vi "ExecutionView(CSM).vi"(7 "Name(\"\" to use uuid)":string="TestStandOI") -> ()   [LabVIEW 2020, in "CSMScript-Engine(Lite).lvlib"]
doc: "------------- lvcsm -------------\n[CSMStates]\nItem 0 = \"Idle\"\nItem 1 = \"CSM Documentation\"\nItem 2 = \"Error Handler\"\nItem 3 = \"VI Reference\"\nItem 4 = \"Critical Error\"\nItem 5 = \"Target Timeout Error\"\nItem 6 = \"Target Error\"\nItem 7 = \"Async Response\"\nItem 8 = \"Response\"\nItem 9 = \"Async Message Posted\"\nItem 10 = \"Initialize Core Data\"\nItem 11 = \"Exit\"\nItem 12 = \"Data: Initialize\"\nItem 13 = \"Data: Get Configuration\"\nItem 14 = \"Data: Get Internal Data\"\nItem 15 = \"Data: Set Configuration\"\nItem 16 = \"Data: Cleanup\"\nItem 17 = \"UI: Initialize\"\nItem 18 = \"UI: Cursor Set\"\nItem 19 = \"UI: Front Panel State\"\nItem 20 = \"Macro: Initialize\"\nItem 21 = \"Macro: Exit\"\nItem 22 = \"TS: Load Sequence\"\nItem 23 = \"TS: Link to Engine\"\nItem 24 = \"TS: Test Started Handler\"\nItem 25 = \"TS: Step Start Handler\"\nItem 26 = \"TS: Step Complete Handler\"\nItem 27 = \"TS: Test Complete Handler\"\nItem 28 = \"Internal: action1\"\nItem 29 = \"Internal: action2\"\n\n[CSMStatus]\nItem 0 = \"Error Occurred@Error Handler\""
uses:
  CSMScript-Engine(Lite).lvlib
  <vilib>/Utility/miscctls.llb/LVRowAndColumnTypeDef.ctl
  Engine/Typedef/Def-StepComplete Event Data.ctl
  49887391-5aaa-4a15-bec5-64cc18cfe9d0.vi
  d29669de-e3bc-4aa1-abb6-bef5024a48d5.vi
  844f5a0a-3cc9-4d1a-ab8e-12611138b1fa.vi
  f99f0b71-739f-43a4-ba27-9b21da8a90fc.vi
  <userlib>/_NEVSTOP/Communicable State Machine(CSM)/_Support/Common/Format Timestamp.vi
  <userlib>/_NEVSTOP/Communicable State Machine(CSM)/AdvanceAPI/CSM - Revert Arguments-Safe String.vi
  <userlib>/_NEVSTOP/Communicable State Machine(CSM)/AdvanceAPI/CSM - Make String Arguments Safe.vi
  <userlib>/_NEVSTOP/Communicable State Machine(CSM)/AdvanceAPI/CSM - Break Down Multiple States String.vi
  <userlib>/_NEVSTOP/Communicable State Machine(CSM)/AdvanceAPI/CSM - Compact Multiple States.vi
  <userlib>/_NEVSTOP/Communicable State Machine(CSM)/_Support/GlobalEvent/GEvt-Generate with Rule Check.vi
  <userlib>/_NEVSTOP/Communicable State Machine(CSM)/_Support/GlobalEvent/Cache-GEvt Refs.vi
  <userlib>/_NEVSTOP/Communicable State Machine(CSM)/AdvanceAPI/CSM - Keywords.vi
  <userlib>/_NEVSTOP/Communicable State Machine(CSM)/_Support/ChangeFlag/FlagInstance-GEvt Refs.vi
  <userlib>/_NEVSTOP/Communicable State Machine(CSM)/_Support/ChangeFlag/ChangeFlag-Read.vi
  <userlib>/_NEVSTOP/Communicable State Machine(CSM)/_Shared/Trim Single-line Text.vi
  <userlib>/_NEVSTOP/Communicable State Machine(CSM)/_Support/ChangeFlag/ChangeFlagDB.vi
  <userlib>/_NEVSTOP/Communicable State Machine(CSM)/_Support/GlobalEvent/FGV-GlobalEventRef(lvlibp).vi
  <userlib>/_NEVSTOP/Communicable State Machine(CSM)/_Support/GlobalEvent/FGV-GlobalEventQueues(lvlibp).vi
  <userlib>/_NEVSTOP/Communicable State Machine(CSM)/_Support/GlobalEvent/GEvt-Valid Subscribers.vi
  <userlib>/_NEVSTOP/Communicable State Machine(CSM)/_Support/GlobalEvent/LogFilter/LogFilter - Check.vi
  <userlib>/_NEVSTOP/Communicable State Machine(CSM)/addons/API-String-Arugments-Support/_Support/Query Data as API String Arguments(variant).vi
  <userlib>/_NEVSTOP/Communicable State Machine(CSM)/addons/API-String-Arugments-Support/_Support/Convert API String Arguments to Data(variant).vi
  resource/global-rc-strings.vi
  <userlib>/_NEVSTOP/Communicable State Machine(CSM)/_Polymophic/CSM - Replace Marks in Messages.vi
  <userlib>/_NEVSTOP/Communicable State Machine(CSM)/_Support/GlobalEvent/LogFilter/LogFilter.lvclass
  <userlib>/_NEVSTOP/Communicable State Machine(CSM)/Communicable State Machine.lvlib
  <userlib>/_NEVSTOP/Communicable State Machine(CSM)/_tool/_ui/csm-ui-support.lvlib
panel:
  in  "Sequence Viewer":i32(listbox)=-1
  out "State History":string="[14:36:06.041] UI: Initialize\r[14:36:06.041] Initialize Core Data\r[14:36:06.041] Data: Initialize\r[14:36:06.041] Macro: Initialize\r"
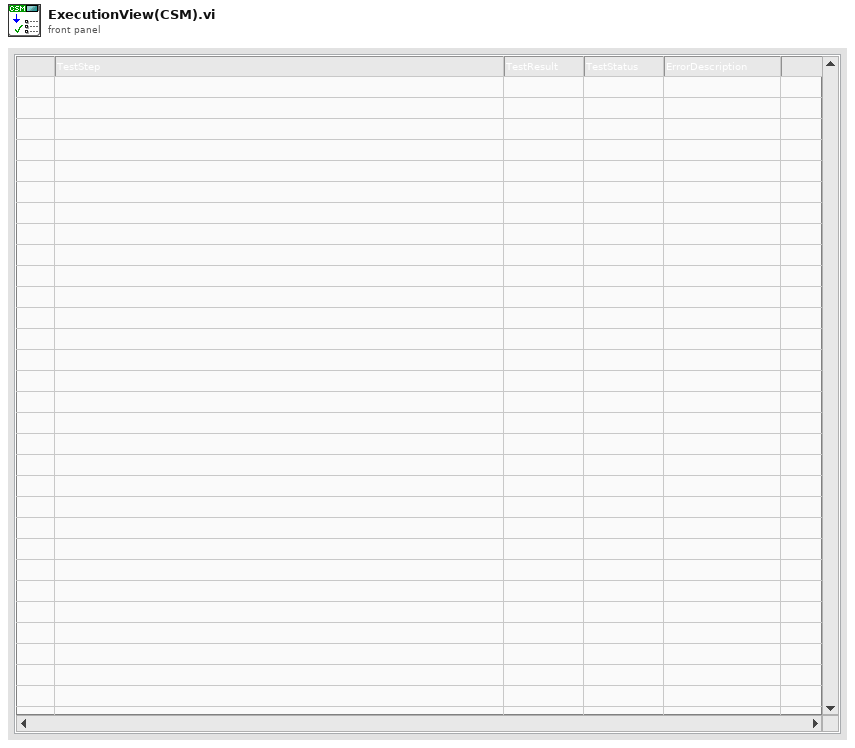
[diagram p1: front panel]
types:
  T1 = enum32{"Invalid", "Standard", "Closed", "Hidden", "Minimized", "Maximized"}
  T2 = enum32{"invalid app kind", "Development System", "Run Time System", "Student Edition", "Embedded LabVIEW", "Evaluation", "Custom"}
  T3 = typedef "LVRowAndColumnTypeDef.ctl" = cluster{"Row":i32, "Column":i32}
  T4 = typedef "CSMScript-Engine(Lite).lvlib/Def-StepComplete Event Data.ctl" = cluster{"index":i32, "Response":string, "error":errorcluster}
  T5 = typedef "Communicable State Machine.lvlib/_CSM_Response Source Message.ctl" = cluster{"‘State":string, "’Arguments":string, "’Error":errorcluster}
  T6 = cluster{"Current VI Reference":refnum<vi>, "Close Panel on Exit?":bool}
  T7 = cluster{"Core":cluster{"Current VI Reference":refnum<vi>, "Close Panel on Exit?":bool}, "Sequence Viewer":refnum<vi>, "ResponseMaxLen":i32}
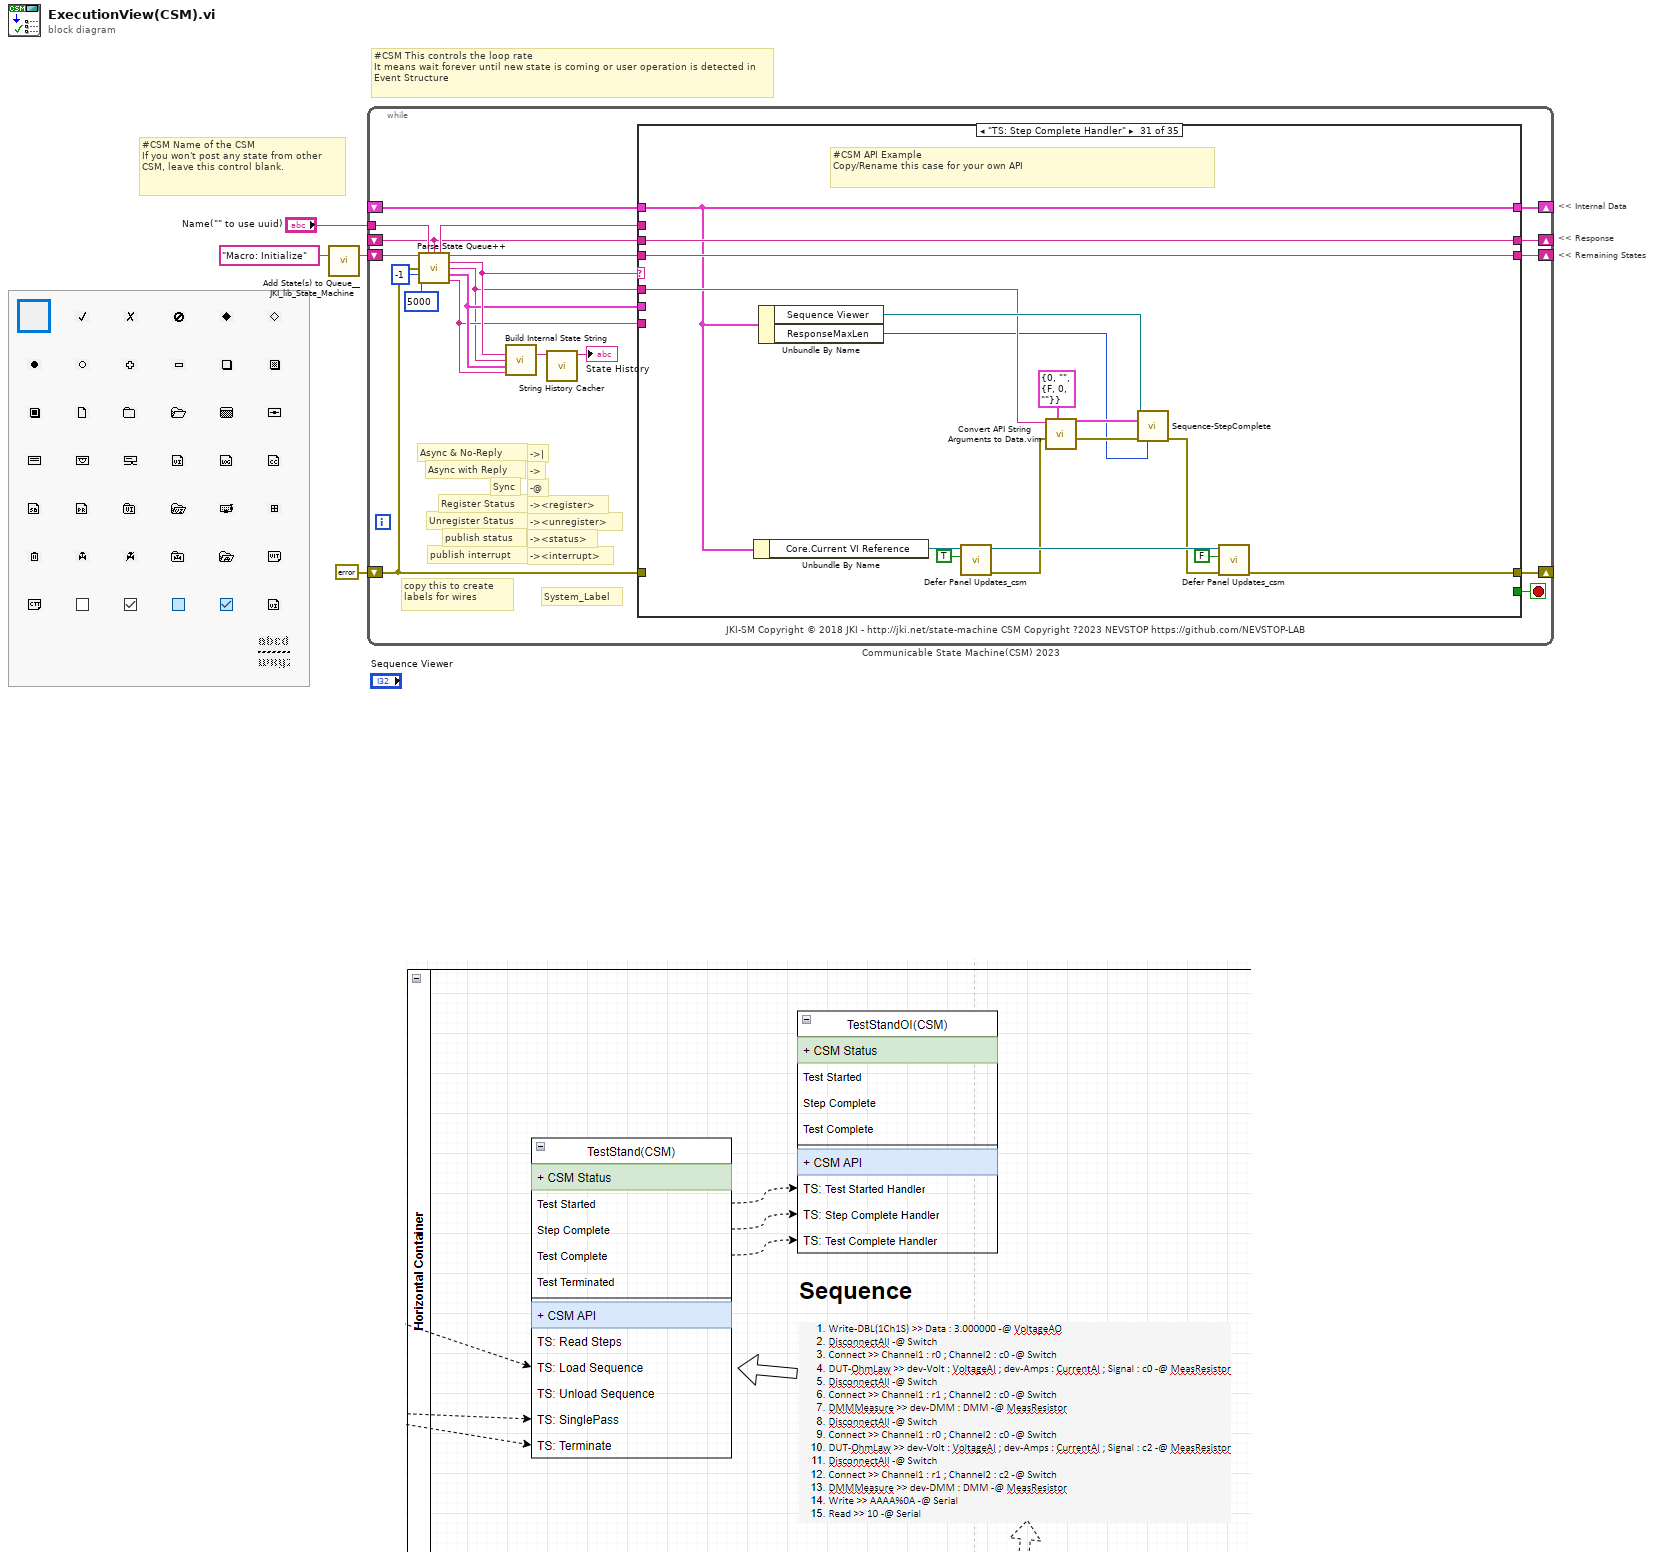
[diagram p0: block diagram]
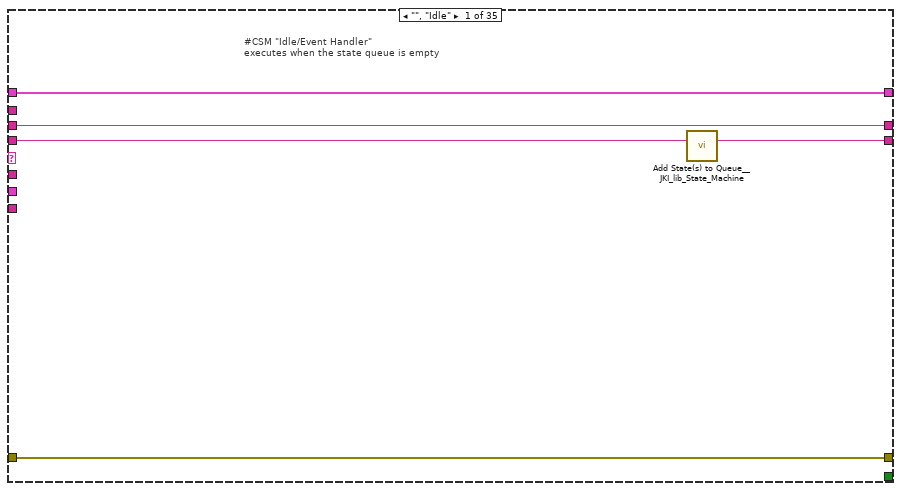
[diagram p2: hidden frame]
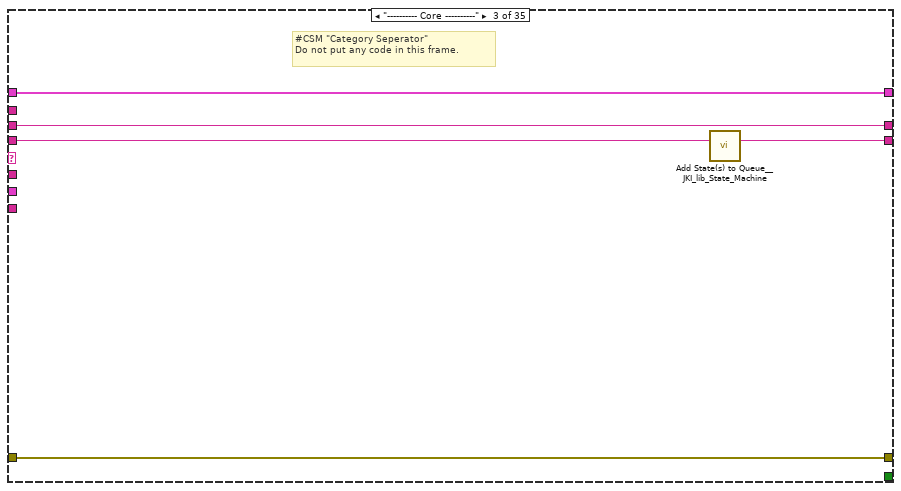
[diagram p4: hidden frame]
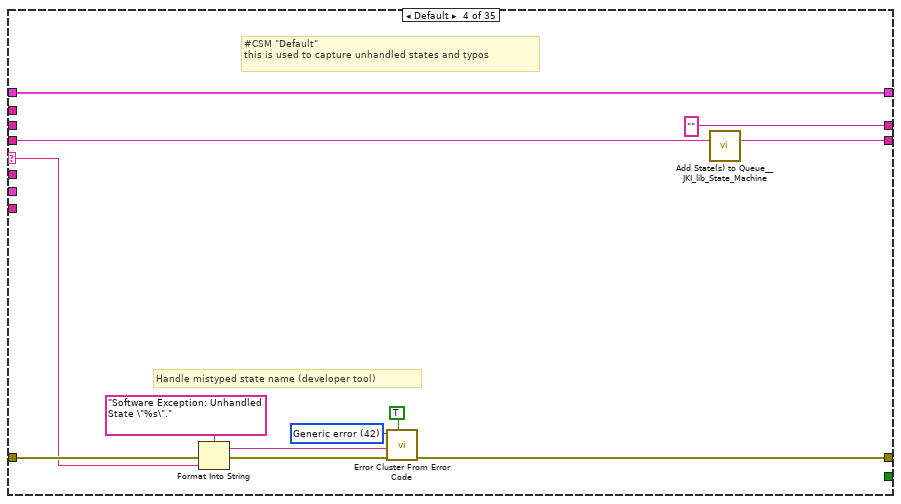
[diagram p5: hidden frame]
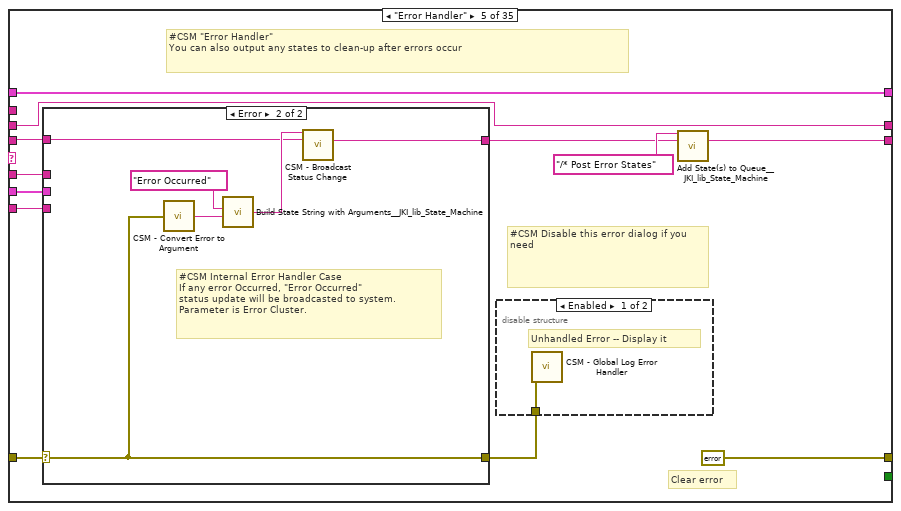
[diagram p6: hidden frame]
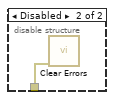
[diagram p7: hidden frame]
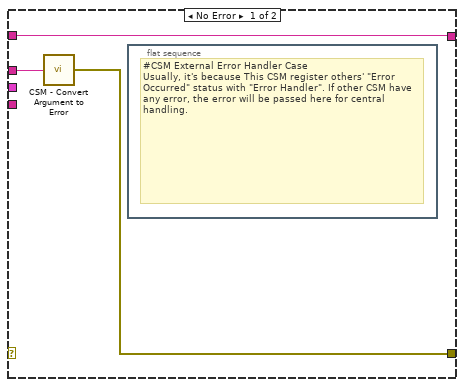
[diagram p8: hidden frame]
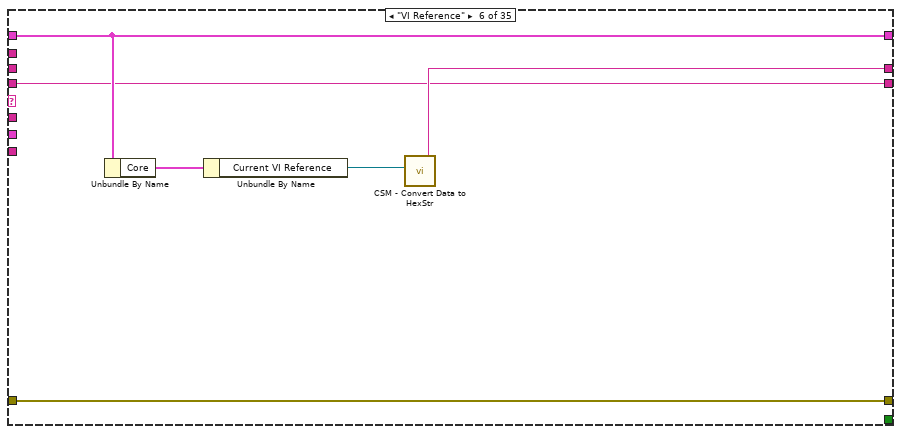
[diagram p9: hidden frame]
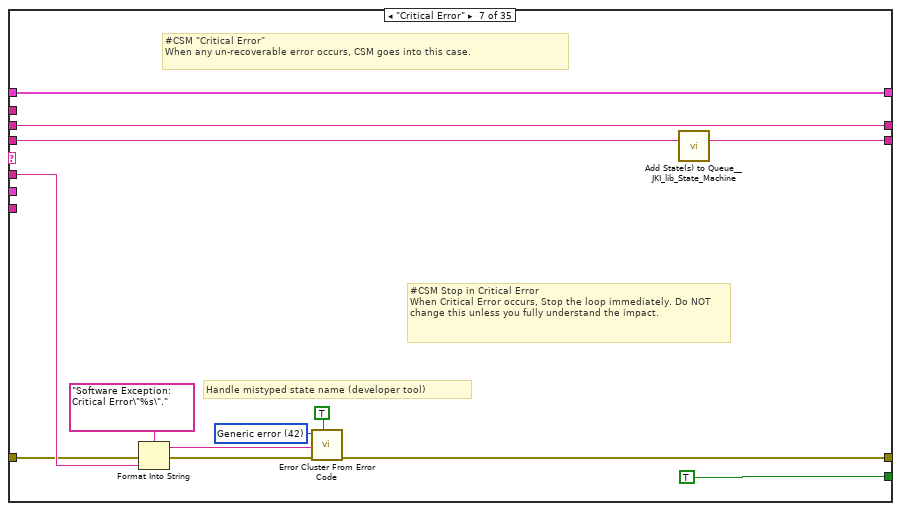
[diagram p10: hidden frame]
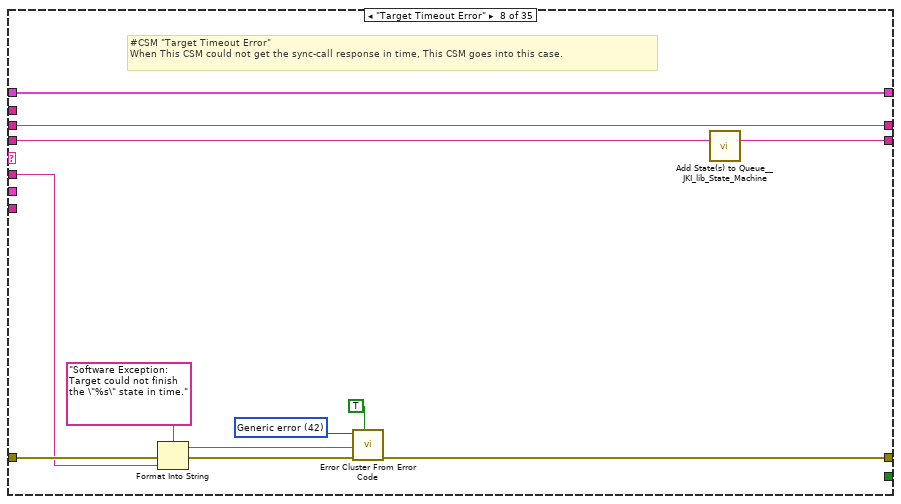
[diagram p11: hidden frame]
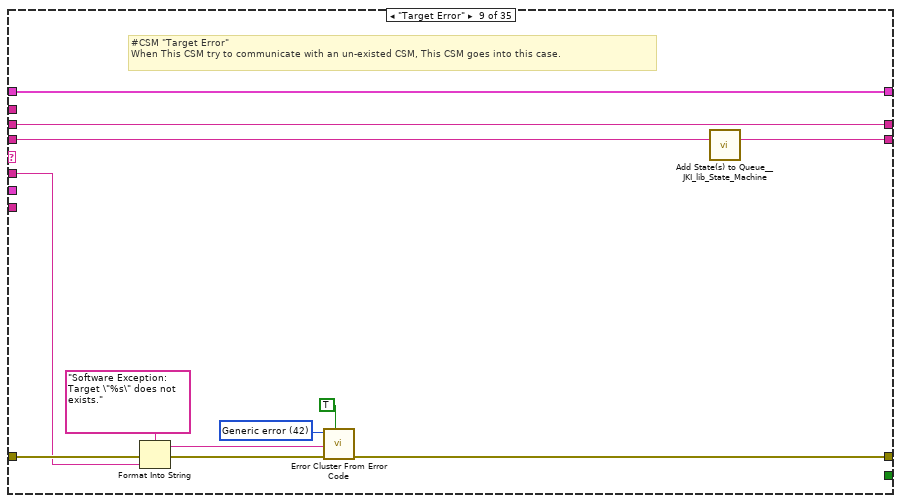
[diagram p12: hidden frame]
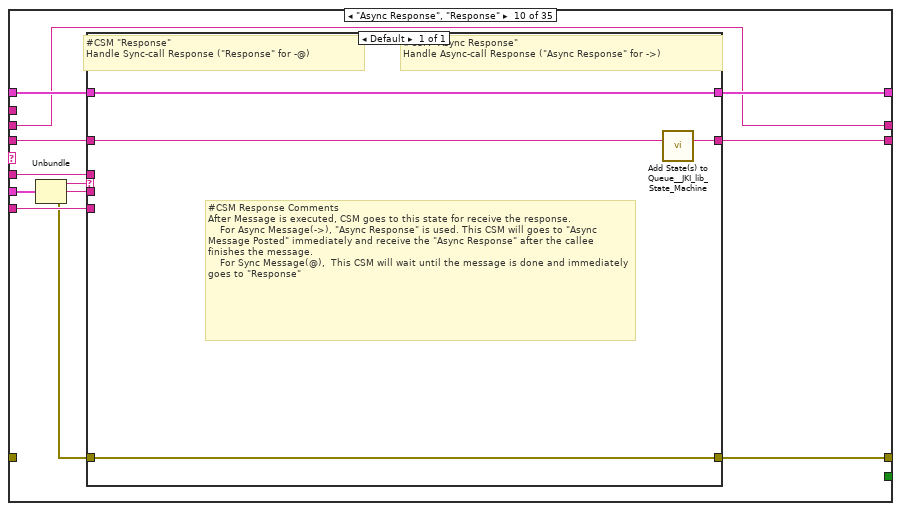
[diagram p13: hidden frame]
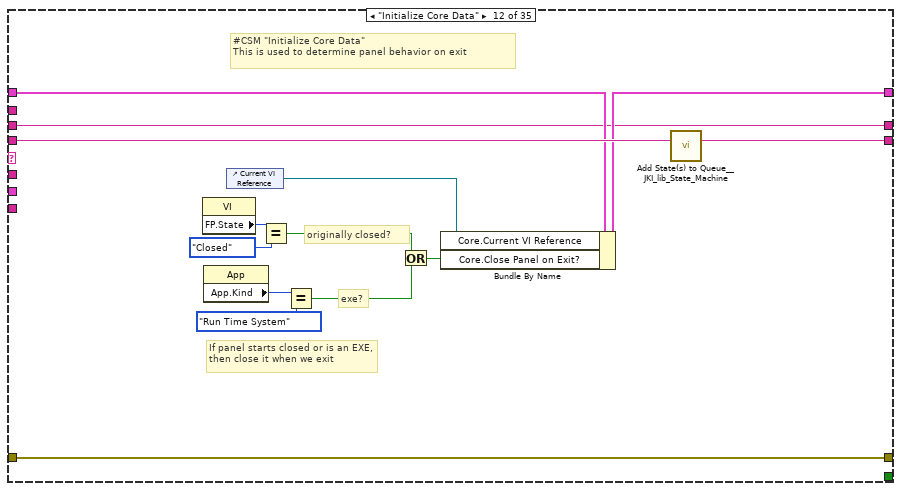
[diagram p15: hidden frame]
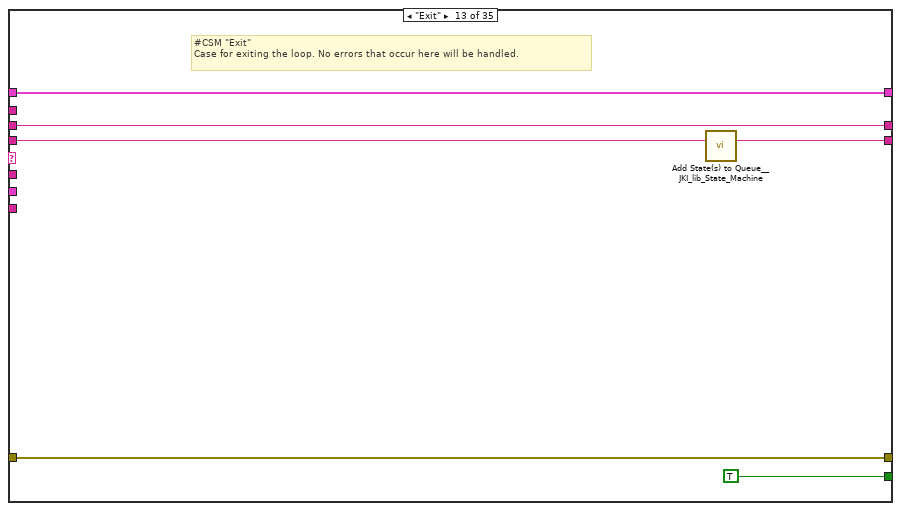
[diagram p16: hidden frame]
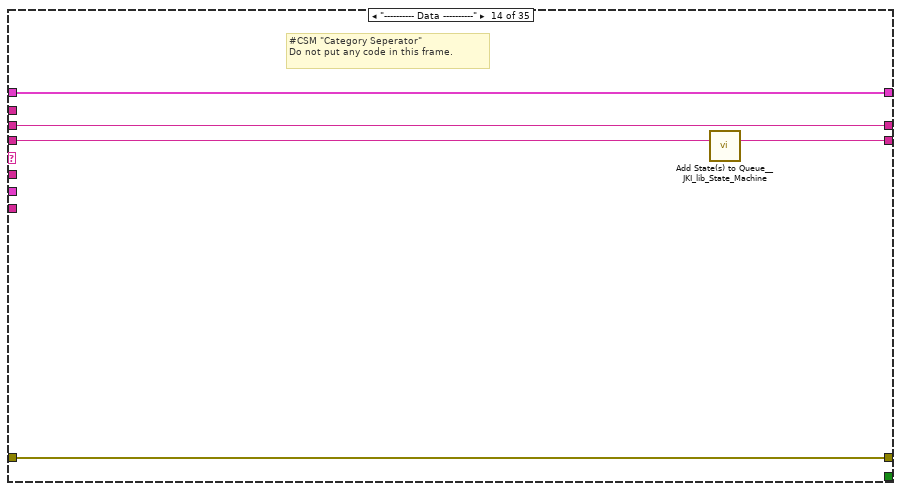
[diagram p17: hidden frame]
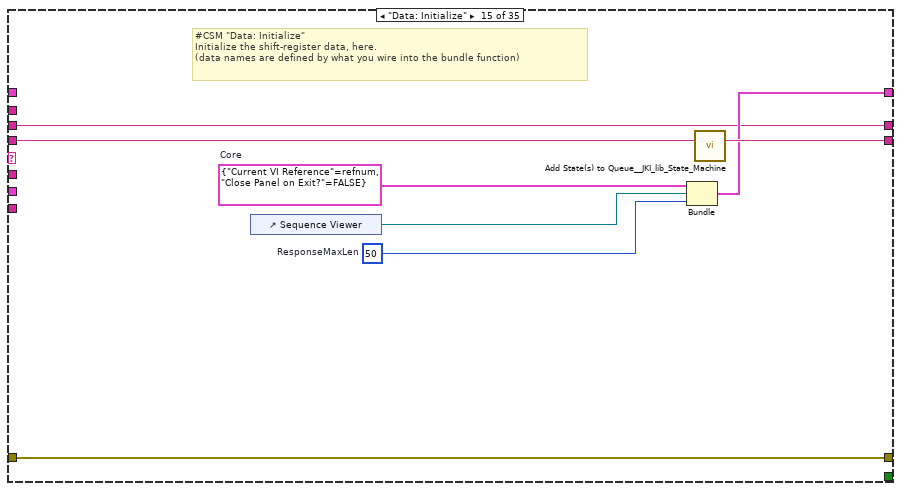
[diagram p18: hidden frame]
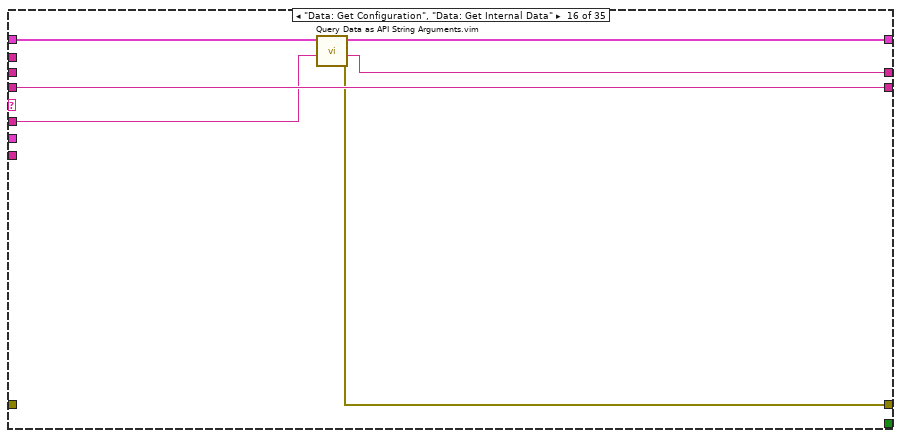
[diagram p19: hidden frame]
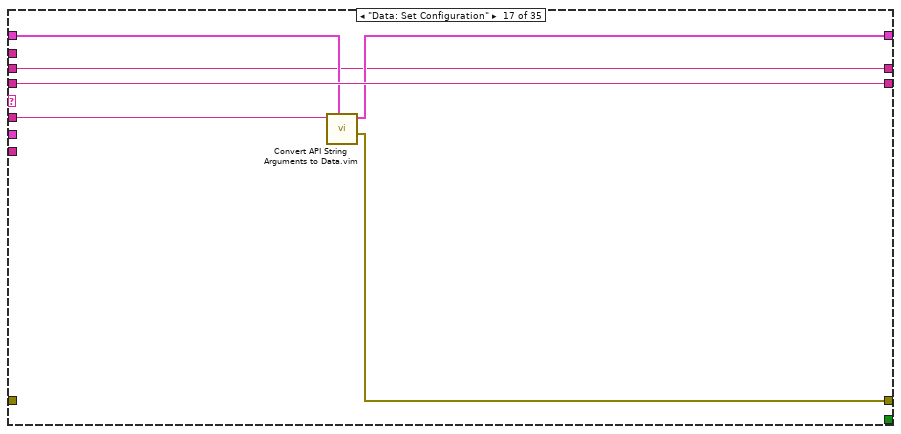
[diagram p20: hidden frame]
diagram:
  # "<< Internal Data"
  # "<< Response"
  # "<< Remaining States"
  # "#CSM Name of the CSM\nIf you won't post any state from other CSM, leave this control blank."
  # "#CSM This controls the loop rate\nIt means wait forever until new state is coming or user operation is detected in Event Structure"
  n1 = call <vilib>:"Add State(s) to Queue__JKI_lib_State_Machine.vi"("State(s) in (\"\")"="Macro: Initialize" ("Init State(\"Macro: Initialize\")")) -> ("States Out"=w1:string)  [unwired: 14 in]
  n2 = while "Communicable State Machine(CSM) 2023" {
    shift-right: [w19] -> _
    shift-left: _ -> [w18]
    shift-right: [w22] -> _
    shift-left: errorcluster {"status"=FALSE, "code"=0, "source"=""} ("error out") -> [w17]
    shift-right: [w21] -> _
    shift-left: w1 -> [w23]
    tunnel: "Name(\"\" to use uuid)" -> [w14]
    shift-right: [w15] -> _
    shift-left: _ -> [w7]
    stop <- w20 stop-if-true
    # "-><interrupt>"
    # "-><status>"
    # "-><unregister>"
    # "-><register>"
    # "-@"
    # "->"
    # "->|"
    # "publish interrupt"
    # "publish status"
    # "Unregister Status"
    # "Register Status"
    # "Sync"
    # "Async with Reply"
    # "Async & No-Reply"
    # "copy this to create labels for wires"
    # "System_Label"
    # "JKI-SM Copyright © 2018 JKI - http://jki.net/state-machine CSM Copyright ?2023 NEVSTOP https://github.com/NEVSTOP-LAB"
    n3 = call <userlib>:"Parse State Queue++.vi"("State Queue"=w23, "Name (\"\" to Use UUID)"=w14, "Response Arguments"=w7, "Previous Error"=w17, "Dequeue (1 ms)"=-1 ("Dequeue Timeout(0ms)"), "Response Timeout (-2 Use Global Settings)"=5000 ("Response Timeout(1000ms)")) -> ("Name Used"=w8:string, "Remaining States"=w24:string, "Current State"=w11:string, "Arguments"=w6:string, "Additional Information"=w10:T5, "Source CSM"=w9:string)  [unwired: 4 in]
    n4 = call <userlib>:"Build Internal State String.vi"("State"=w11, "Arguments (\"\")"=w6, "Additional Information"=w10, "Source (\"\")"=w9) -> ("State With Arguments"=w12:string)  [unwired: 11 in]
    n5 = call <userlib>:"String History Cacher.vi"("String"=w12) -> ("String Cache"=→"State History":string)  [unwired: 10 in]
    n6 = case shown="\"TS: Step Complete Handler\"" w11 {
      selector: w11 -> [_ _ _ w40 _ _ _ _ _ _ _ _ _ _ _ _ _ _ _ _ _ _ _ _ _ _ _ _ _ _ _ _ _ _ _]
      tunnel: w24 -> [w26 w33 w38 w44 w56 w75 w91 w99 w111 w127 w135 w150 w156 w161 w169 w175 w181 w188 w193 w220 w227 w243 w313 w319 w331 w334 w350 w354 w370 w385 w401 w404 w410 w415 w420]
      tunnel: w6 -> [_ _ _ _ w54 _ w84 w95 w107 w121 _ _ _ _ _ w172 w180 _ _ _ w222 w237 _ _ _ _ w344 w351 _ w382 w397 _ _ _ _]
      tunnel: w18 -> [w27 w32 w35 w42 w61 w79 w92 w97 w109 w125 w134 w143 w154 w158 _ w174 w179 w183 w190 w218 w225 w239 w310 w316 w328 w333 w348 w356 w359 w374 w386 w403 w407 w412 w417]
      tunnel: [w28 w31 w36 w46 errorcluster {"status"=FALSE, "code"=0, "source"=""} ("error out") w74 w81 w94 w106 w124 w136 w147 w153 w159 w166 w170 w177 w184 w191 w203 w223 w240 w311 w317 w329 w335 w341 w357 w361 w375 w387 w405 w408 w413 w418] -> w22
      tunnel: w17 -> [w28 w31 w36 w45 w60 w74 w82 w100 w112 _ w136 w147 w153 w159 w166 _ _ w185 w191 w215 w224 w241 w311 w317 w329 w335 _ w357 w360 _ _ w405 w408 w413 w418]
      tunnel: [w29 w33 w37 w43 w58 w75 w90 w98 w110 w128 w135 w149 w155 w160 w168 w175 w181 w187 w192 w219 w226 w242 w312 w318 w330 w334 w349 w355 w369 w385 w401 w404 w409 w414 w419] -> w21
      tunnel: [_ _ _ _ _ _ TRUE _ _ _ _ _ TRUE _ _ _ _ _ _ _ _ _ _ _ _ _ _ _ _ _ _ _ _ _ _] -> w20
      tunnel: [w27 w32 w35 w42 w61 w79 w92 w97 w109 w126 w134 w148 w154 w158 w167 w173 w178 w183 w190 w218 w225 w239 w310 w316 w328 w333 w348 w356 w359 w374 w386 w403 w407 w412 w417] -> w19
      tunnel: w9 -> [_ _ _ _ w53 _ _ _ _ w122 _ _ _ _ _ _ _ _ _ _ _ _ _ _ _ _ _ _ _ _ _ _ _ _ _]
      tunnel: w10 -> [_ _ _ _ w52 _ _ _ _ w123 _ _ _ _ _ _ _ _ _ _ _ _ _ _ _ _ _ _ _ _ _ _ _ _ _]
      tunnel: [w25 w30 w34 "" w51 w76 w80 w93 w105 w117 w133 w137 w151 w157 w163 w171 w176 w182 w189 w200 w221 w236 w309 w314 w320 w332 w343 _ w368 w380 w395 w402 w406 w411 w416] -> w15
      tunnel: w8 -> [_ _ _ _ _ _ _ _ _ _ _ _ _ _ _ _ _ _ _ _ _ _ _ _ _ _ _ _ _ _ _ _ _ _ _]
      tunnel: w7 -> [w25 w30 w34 _ w51 _ w80 w93 w105 w117 w133 w137 w151 w157 w163 _ w176 w182 w189 w200 w221 w236 w309 w314 w320 w332 w343 _ w368 w380 w395 w402 w406 w411 w416]
      frame "", "Idle" {
        # "#CSM \"Idle/Event Handler\"\nexecutes when the state queue is empty"
        n7 = call <vilib>:"Add State(s) to Queue__JKI_lib_State_Machine.vi"("State(s) in (\"\")"=w26) -> ("States Out"=w29:string)  [unwired: 14 in]
      }
      frame "CSM Documentation" {
        # "CSM Documentation"
        # "#CSM State Syntax\n\n// Comment line, all text to the right of “//” will be ignored\n// Local Message Example\nDoSth: DoA >> Arguments\n\n// Sync Call Example\nAPI: xxxx >> Arguments -@ TargetModule\n\n// Async Call Example\nAPI: xxxx >> Arguments -> TargetModule\n\n// Async Call without Reply Example\nAPI: xxxx >> Arguments ->| TargetModule\n\n// Broadcast normal status:\nStatus >> StatusArguments  -><status>\n\n// Broadcast Interrupt status:\nInterrupt >> StatusArguments  -><interrupt>\n\n// Register Source Module's status to Handler Module\nStatus@Source Module >> Handler Module@Handler Module -><register>\n\n// Unegister Source Module's status\nStatus@Source Module >> Handler Module -><unregister>"
        # "#CSM README FIRST\n\nCSM is a LabVIEW application framework that builds upon JKI State Machine (JKISM). It follows the pattern of JKISM and extends the keywords to describe message communication between CSM modules, including concepts such as Sync-Message, Async-Message, Subscription/Unsubscription of status - essential elements for creating reusable code modules. \n\nFor more information, please visit the CSM wiki: https://github.com/NEVSTOP-LAB/JKI-State-Machine-Plus-Plus/wiki\n\nFor instructions on JKI State Machine, visit: \n    http://jki.net/state-machine/\nFor information about CSM, visit: \n    https://github.com/NEVSTOP-LAB"
        # "#CSM \"Documentation\"\nCase for holding CSM Documenation"
      }
      frame "---------- Core ----------" {
        # "#CSM \"Category Seperator\"\nDo not put any code in this frame."
        n8 = call <vilib>:"Add State(s) to Queue__JKI_lib_State_Machine.vi"("State(s) in (\"\")"=w38) -> ("States Out"=w37:string)  [unwired: 14 in]
      }
      frame Default {
        w49 = 42 items=["No error", "Argument error", "Memory is full", "Out of zone", "End of file", "File already open", "Generic file I/O error", "File not found", "File permission error", "Disk is full", "Duplicate path", "Too many files open", "System feature not enabled", "Resource file not found", "Cannot add resource", "Resource not found", "Image not found", "Image memory error", "Pen does not exist", "Config type invalid", "Config token not found", "Config parse error", "Config memory error", "Bad external code format", "Bad external code offset", "External code not present", "Null window", "Destroy window error", "Null menu", "Print aborted", "Bad print record", "Print driver error", "Windows error during printing", "Memory error during printing", "Print dialog error", "Generic print error", "Invalid device refnum", "Device not found", "Device parameter error", "Device unit error", "Cannot open device", "Device call aborted", "Generic error", "Cancelled by user", "Object ID too low", "Object ID too high", "Object not in heap", "Unknown heap", "Unknown object (invalid DefProc)", "Unknown object (DefProc not in table)", "Message out of range", "Invalid (null) method", "Unknown message", "Manager call not supported", "Bad address", "Network operation in progress", "Network operation timed out", "Connection is busy", "Network attribute not supported", "Network error", "Address in use", "System out of memory", "Connection aborted", "Connection refused", "Not connected", "Already connected", "Connection closed", "Initialization error (interapplication manager)", "Bad occurrence", "Wait on unbound occurrence handler", "Occurrence queue overflow", "Datalog type conflict", "Unused", "Unrecognized type (interapplication manager)", "Memory corrupt", "Failed to make temporary DLL", "Old CIN version", "Drag socket not found", "Failed to load drop-object", "Failed to register OLE object", "Failed to release OLE object", "Format specifier type mismatch", "Unknown format specifier", "Too few format specifiers", "Too many format specifiers", "Scan failed", "Newer CIN version", "Error converting to variant", "Runtime menu error", "Password tampered", "Variant attribute not found", "Incompatible variant data type", "Event data is not available", "Event Store is not present", "Occurrence is not found", "Event Queue is not created", "Event info is not available", "Refnum passed is NULL", "Error retrieving Class GUID", "Error retrieving CoClass GUID", "Error retrieving TypeLib GUID.", "Bad built application magic bytes.", "Specific driver is different from the specific driver associated with the Logical Name.", "There is no session opened to the class driver.", "Max Error", "MAX - Error with config objects", "MAX - Error loading configuration", "MAX - Group not supported"]
        # "#CSM \"Default\"\nthis is used to capture unhandled states and typos"
        # "Handle mistyped state name (developer tool)"
        n9 = Format Into String(format string="Software Exception: Unhandled State \"%s\"." ("message"), error in=w45, w40) -> (resulting string=w48:string, error out=w47:errorcluster)  [unwired: 1 in]
        n10 = call <vilib>:"Error Cluster From Error Code.vi"("show call chain? (False)"=TRUE, "error in (no error)"=w47, "error message (\"\")"=w48, "error code (0)"=w49) -> ("error out"=w46:errorcluster)  [unwired: 5 in]
        n11 = call <vilib>:"Add State(s) to Queue__JKI_lib_State_Machine.vi"("State(s) in (\"\")"=w44) -> ("States Out"=w43:string)  [unwired: 14 in]
      }
      frame "Error Handler" {
        # "#CSM Disable this error dialog if you need"
        # "#CSM \"Error Handler\"\nYou can also output any states to clean-up after errors occur"
        # "Clear error"
        n12 = case shown="Error" w60 {
          selector: w60 -> [_ w68]
          tunnel: [w66 w70] -> w57
          tunnel: w56 -> [w66 w69]
          tunnel: [w65 w68] -> w55
          tunnel: w54 -> [w67 _]
          tunnel: w53 -> [_ _]
          tunnel: w52 -> [_ _]
          frame No Error {
            n13 = call <userlib>:"CSM - Convert Argument to Error.vi"("Argument"=w67) -> ("Error"=w65:errorcluster)  [unwired: 4 in]
            n14 = flat-sequence {
              frame #0 {
                # "#CSM External Error Handler Case\nUsually, it's because This CSM register others' \"Error Occurred\" status with \"Error Handler\". If other CSM have any error, the error will be passed here for central handling."
              }
            }
          }
          frame Error {
            # "#CSM Internal Error Handler Case \nIf any error Occurred, \"Error Occurred\" \nstatus update will be broadcasted to system.\nParameter is Error Cluster."
            n15 = call <userlib>:"CSM - Convert Error to Argument.vi"("Error"=w68) -> ("Argument"=w72:string)  [unwired: 4 in]
            n16 = call <vilib>:"Build State String with Arguments__JKI_lib_State_Machine.vi"("Arguments (\"\")"=w72, "State"="Error Occurred" ("Status with Arguments")) -> ("State with Arguments"=w71:string)  [unwired: 4 in]
            n17 = call <userlib>:"CSM - Broadcast Status Change.vi"("Status With Arguments"=w71, "State Queue"=w69) -> ("Remaining States"=w70:string)  [unwired: 13 in]
          }
        }
        n18 = disable-structure shown="Enabled" {
          disable-tunnel: w55 -> [w63 w64]
          frame Enabled {
            # "Unhandled Error -- Display it"
            n19 = call <userlib>:"CSM - Global Log Error Handler.vi"("Error In"=w63) -> ()  [unwired: 10 in, 1 out]
          }
          frame Disabled {
            n20 = call <vilib>:"Clear Errors.vi"("error in (no error)"=w64) -> ()  [unwired: 5 in, 2 out]
          }
        }
        n21 = call <vilib>:"Add State(s) to Queue__JKI_lib_State_Machine.vi"("State(s) in Front (\"\")"="/* Post Error States", "State(s) in (\"\")"=w57) -> ("States Out"=w58:string)  [unwired: 13 in]
      }
      frame "VI Reference" {
        n22 = Unbundle By Name(w79) -> ("Core"=w78:T6)
        n23 = Unbundle By Name(w78) -> ("Current VI Reference"=w77:refnum<vi>)
        n24 = call <userlib>:"CSM - Convert Data to HexStr.vi"("Variant"=w77) -> ("HEX String (0-9,A-F)"=w76:string)  [unwired: 8 in]
      }
      frame "Critical Error" {
        w88 = 42 items=["No error", "Argument error", "Memory is full", "Out of zone", "End of file", "File already open", "Generic file I/O error", "File not found", "File permission error", "Disk is full", "Duplicate path", "Too many files open", "System feature not enabled", "Resource file not found", "Cannot add resource", "Resource not found", "Image not found", "Image memory error", "Pen does not exist", "Config type invalid", "Config token not found", "Config parse error", "Config memory error", "Bad external code format", "Bad external code offset", "External code not present", "Null window", "Destroy window error", "Null menu", "Print aborted", "Bad print record", "Print driver error", "Windows error during printing", "Memory error during printing", "Print dialog error", "Generic print error", "Invalid device refnum", "Device not found", "Device parameter error", "Device unit error", "Cannot open device", "Device call aborted", "Generic error", "Cancelled by user", "Object ID too low", "Object ID too high", "Object not in heap", "Unknown heap", "Unknown object (invalid DefProc)", "Unknown object (DefProc not in table)", "Message out of range", "Invalid (null) method", "Unknown message", "Manager call not supported", "Bad address", "Network operation in progress", "Network operation timed out", "Connection is busy", "Network attribute not supported", "Network error", "Address in use", "System out of memory", "Connection aborted", "Connection refused", "Not connected", "Already connected", "Connection closed", "Initialization error (interapplication manager)", "Bad occurrence", "Wait on unbound occurrence handler", "Occurrence queue overflow", "Datalog type conflict", "Unused", "Unrecognized type (interapplication manager)", "Memory corrupt", "Failed to make temporary DLL", "Old CIN version", "Drag socket not found", "Failed to load drop-object", "Failed to register OLE object", "Failed to release OLE object", "Format specifier type mismatch", "Unknown format specifier", "Too few format specifiers", "Too many format specifiers", "Scan failed", "Newer CIN version", "Error converting to variant", "Runtime menu error", "Password tampered", "Variant attribute not found", "Incompatible variant data type", "Event data is not available", "Event Store is not present", "Occurrence is not found", "Event Queue is not created", "Event info is not available", "Refnum passed is NULL", "Error retrieving Class GUID", "Error retrieving CoClass GUID", "Error retrieving TypeLib GUID.", "Bad built application magic bytes.", "Specific driver is different from the specific driver associated with the Logical Name.", "There is no session opened to the class driver.", "Max Error", "MAX - Error with config objects", "MAX - Error loading configuration", "MAX - Group not supported"]
        # "#CSM \"Critical Error\"\nWhen any un-recoverable error occurs, CSM goes into this case."
        # "#CSM Stop in Critical Error\nWhen Critical Error occurs, Stop the loop immediately. Do NOT change this unless you fully understand the impact."
        # "Handle mistyped state name (developer tool)"
        n25 = Format Into String(format string="Software Exception: Critical Error\"%s\"." ("message"), error in=w82, w84) -> (resulting string=w87:string, error out=w86:errorcluster)  [unwired: 1 in]
        n26 = call <vilib>:"Error Cluster From Error Code.vi"("show call chain? (False)"=TRUE, "error in (no error)"=w86, "error message (\"\")"=w87, "error code (0)"=w88) -> ("error out"=w81:errorcluster)  [unwired: 5 in]
        n27 = call <vilib>:"Add State(s) to Queue__JKI_lib_State_Machine.vi"("State(s) in (\"\")"=w91) -> ("States Out"=w90:string)  [unwired: 14 in]
      }
      frame "Target Timeout Error" {
        w103 = 42 items=["No error", "Argument error", "Memory is full", "Out of zone", "End of file", "File already open", "Generic file I/O error", "File not found", "File permission error", "Disk is full", "Duplicate path", "Too many files open", "System feature not enabled", "Resource file not found", "Cannot add resource", "Resource not found", "Image not found", "Image memory error", "Pen does not exist", "Config type invalid", "Config token not found", "Config parse error", "Config memory error", "Bad external code format", "Bad external code offset", "External code not present", "Null window", "Destroy window error", "Null menu", "Print aborted", "Bad print record", "Print driver error", "Windows error during printing", "Memory error during printing", "Print dialog error", "Generic print error", "Invalid device refnum", "Device not found", "Device parameter error", "Device unit error", "Cannot open device", "Device call aborted", "Generic error", "Cancelled by user", "Object ID too low", "Object ID too high", "Object not in heap", "Unknown heap", "Unknown object (invalid DefProc)", "Unknown object (DefProc not in table)", "Message out of range", "Invalid (null) method", "Unknown message", "Manager call not supported", "Bad address", "Network operation in progress", "Network operation timed out", "Connection is busy", "Network attribute not supported", "Network error", "Address in use", "System out of memory", "Connection aborted", "Connection refused", "Not connected", "Already connected", "Connection closed", "Initialization error (interapplication manager)", "Bad occurrence", "Wait on unbound occurrence handler", "Occurrence queue overflow", "Datalog type conflict", "Unused", "Unrecognized type (interapplication manager)", "Memory corrupt", "Failed to make temporary DLL", "Old CIN version", "Drag socket not found", "Failed to load drop-object", "Failed to register OLE object", "Failed to release OLE object", "Format specifier type mismatch", "Unknown format specifier", "Too few format specifiers", "Too many format specifiers", "Scan failed", "Newer CIN version", "Error converting to variant", "Runtime menu error", "Password tampered", "Variant attribute not found", "Incompatible variant data type", "Event data is not available", "Event Store is not present", "Occurrence is not found", "Event Queue is not created", "Event info is not available", "Refnum passed is NULL", "Error retrieving Class GUID", "Error retrieving CoClass GUID", "Error retrieving TypeLib GUID.", "Bad built application magic bytes.", "Specific driver is different from the specific driver associated with the Logical Name.", "There is no session opened to the class driver.", "Max Error", "MAX - Error with config objects", "MAX - Error loading configuration", "MAX - Group not supported"]
        # "#CSM \"Target Timeout Error\"\nWhen This CSM could not get the sync-call response in time, This CSM goes into this case."
        n28 = Format Into String(format string="Software Exception: Target could not finish the \"%s\" state in time." ("message"), error in=w100, w95) -> (resulting string=w102:string, error out=w101:errorcluster)  [unwired: 1 in]
        n29 = call <vilib>:"Error Cluster From Error Code.vi"("show call chain? (False)"=TRUE, "error in (no error)"=w101, "error message (\"\")"=w102, "error code (0)"=w103) -> ("error out"=w94:errorcluster)  [unwired: 5 in]
        n30 = call <vilib>:"Add State(s) to Queue__JKI_lib_State_Machine.vi"("State(s) in (\"\")"=w99) -> ("States Out"=w98:string)  [unwired: 14 in]
      }
      frame "Target Error" {
        w115 = 42 items=["No error", "Argument error", "Memory is full", "Out of zone", "End of file", "File already open", "Generic file I/O error", "File not found", "File permission error", "Disk is full", "Duplicate path", "Too many files open", "System feature not enabled", "Resource file not found", "Cannot add resource", "Resource not found", "Image not found", "Image memory error", "Pen does not exist", "Config type invalid", "Config token not found", "Config parse error", "Config memory error", "Bad external code format", "Bad external code offset", "External code not present", "Null window", "Destroy window error", "Null menu", "Print aborted", "Bad print record", "Print driver error", "Windows error during printing", "Memory error during printing", "Print dialog error", "Generic print error", "Invalid device refnum", "Device not found", "Device parameter error", "Device unit error", "Cannot open device", "Device call aborted", "Generic error", "Cancelled by user", "Object ID too low", "Object ID too high", "Object not in heap", "Unknown heap", "Unknown object (invalid DefProc)", "Unknown object (DefProc not in table)", "Message out of range", "Invalid (null) method", "Unknown message", "Manager call not supported", "Bad address", "Network operation in progress", "Network operation timed out", "Connection is busy", "Network attribute not supported", "Network error", "Address in use", "System out of memory", "Connection aborted", "Connection refused", "Not connected", "Already connected", "Connection closed", "Initialization error (interapplication manager)", "Bad occurrence", "Wait on unbound occurrence handler", "Occurrence queue overflow", "Datalog type conflict", "Unused", "Unrecognized type (interapplication manager)", "Memory corrupt", "Failed to make temporary DLL", "Old CIN version", "Drag socket not found", "Failed to load drop-object", "Failed to register OLE object", "Failed to release OLE object", "Format specifier type mismatch", "Unknown format specifier", "Too few format specifiers", "Too many format specifiers", "Scan failed", "Newer CIN version", "Error converting to variant", "Runtime menu error", "Password tampered", "Variant attribute not found", "Incompatible variant data type", "Event data is not available", "Event Store is not present", "Occurrence is not found", "Event Queue is not created", "Event info is not available", "Refnum passed is NULL", "Error retrieving Class GUID", "Error retrieving CoClass GUID", "Error retrieving TypeLib GUID.", "Bad built application magic bytes.", "Specific driver is different from the specific driver associated with the Logical Name.", "There is no session opened to the class driver.", "Max Error", "MAX - Error with config objects", "MAX - Error loading configuration", "MAX - Group not supported"]
        # "#CSM \"Target Error\"\nWhen This CSM try to communicate with an un-existed CSM, This CSM goes into this case."
        n31 = Format Into String(format string="Software Exception: Target \"%s\" does not exists." ("message"), error in=w112, w107) -> (resulting string=w114:string, error out=w113:errorcluster)  [unwired: 1 in]
        n32 = call <vilib>:"Error Cluster From Error Code.vi"("show call chain? (False)"=TRUE, "error in (no error)"=w113, "error message (\"\")"=w114, "error code (0)"=w115) -> ("error out"=w106:errorcluster)  [unwired: 5 in]
        n33 = call <vilib>:"Add State(s) to Queue__JKI_lib_State_Machine.vi"("State(s) in (\"\")"=w111) -> ("States Out"=w110:string)  [unwired: 14 in]
      }
      frame "Async Response", "Response" {
        # "#CSM \"Async Response\"\nHandle Async-call Response (\"Async Response\" for ->)"
        # "#CSM \"Response\"\nHandle Sync-call Response (\"Response\" for -@)"
        n34 = Unbundle(w123) -> ("‘State"=w120:string, "’Arguments"=w119:string, "’Error"=w118:errorcluster)
        n35 = case shown="Default" w120 {
          tunnel: [w129] -> w128
          tunnel: w127 -> [w130]
          tunnel: [w132] -> w126
          tunnel: w125 -> [w132]
          tunnel: [w131] -> w124
          tunnel: w118 -> [w131]
          tunnel: w122 -> [_]
          tunnel: w121 -> [_]
          tunnel: w119 -> [_]
          frame Default {
            # "#CSM Response Comments\nAfter Message is executed, CSM goes to this state for receive the response.\n    For Async Message(->), \"Async Response\" is used. This CSM will goes to \"Async Message Posted\" immediately and receive the \"Async Response\" after the callee finishes the message.\n    For Sync Message(@),  This CSM will wait until the message is done and immediately goes to \"Response\""
            n36 = call <vilib>:"Add State(s) to Queue__JKI_lib_State_Machine.vi"("State(s) in (\"\")"=w130) -> ("States Out"=w129:string)  [unwired: 14 in]
          }
        }
      }
      frame "Async Message Posted" {
        # "#CSM \"Async Message Posted\"\nAfter Async Message is posted (-> or ->| ), CSM goes to this state for post-action.\nYou can use Argument - State to tell which Async Message is called."
      }
      frame "Initialize Core Data" {
        # "#CSM \"Initialize Core Data\"\nThis is used to determine panel behavior on exit"
        # "originally closed?"
        # "exe?"
        # "If panel starts closed or is an EXE, then close it when we exit"
        n37 = property class="VI"() -> ("FP.State"=w140:T1)  [unwired: 2 in, 2 out]
        n38 = property class="App"() -> ("App.Kind"=w146:T2)  [unwired: 2 in, 2 out]
        n39 = control-ref of="Current VI Reference"() -> (w141:refnum<vi>)
        n40 = Equal?(x=w140, y=T1."Closed" ("Front Panel Window:State")) -> (x = y?=w138:bool)
        n41 = Equal?(x=w146, y=T2."Run Time System" ("Application:Kind")) -> (x = y?=w144:bool)
        n42 = Or(x=w138, y=w144) -> (x .or. y?=w142:bool)
        n43 = Bundle By Name(cluster=w143, "Core.Current VI Reference"=w141, "Core.Close Panel on Exit?"=w142) -> (w148:T7)
        n44 = call <vilib>:"Add State(s) to Queue__JKI_lib_State_Machine.vi"("State(s) in (\"\")"=w150) -> ("States Out"=w149:string)  [unwired: 14 in]
      }
      frame "Exit" {
        # "#CSM \"Exit\"\nCase for exiting the loop. No errors that occur here will be handled."
        n45 = call <vilib>:"Add State(s) to Queue__JKI_lib_State_Machine.vi"("State(s) in (\"\")"=w156) -> ("States Out"=w155:string)  [unwired: 14 in]
      }
      frame "---------- Data ----------" {
        # "#CSM \"Category Seperator\"\nDo not put any code in this frame."
        n46 = call <vilib>:"Add State(s) to Queue__JKI_lib_State_Machine.vi"("State(s) in (\"\")"=w161) -> ("States Out"=w160:string)  [unwired: 14 in]
      }
      frame "Data: Initialize" {
        w162 = 50  # ResponseMaxLen
        w165 = T6 {"Current VI Reference"=refnum, "Close Panel on Exit?"=FALSE}  # Core
        # "#CSM \"Data: Initialize\"\nInitialize the shift-register data, here.\n(data names are defined by what you wire into the bundle function)"
        n47 = control-ref of="Sequence Viewer"() -> (w164:refnum<vi>)
        n48 = Bundle("Core"=w165, "Sequence Viewer"=w164, "ResponseMaxLen"=w162) -> (w167:T7)  [unwired: 1 in]
        n49 = call <vilib>:"Add State(s) to Queue__JKI_lib_State_Machine.vi"("State(s) in (\"\")"=w169) -> ("States Out"=w168:string)  [unwired: 14 in]
      }
      frame "Data: Get Configuration", "Data: Get Internal Data" {
        n50 = call "Query Data as API String Arguments.vim"("Name"=w172, "Cluster Data"=w174) -> ("error"=w170:errorcluster, "API String"=w171:string, "Cluster Data (dup)"=w173:T7)  [unwired: 7 in]
      }
      frame "Data: Set Configuration" {
        n51 = call "Convert API String Arguments to Data.vim"("Reference Type"=w179, "API String"=w180) -> ("error out"=w177:errorcluster, "Data"=w178:T7)  [unwired: 6 in]
      }
      frame "Data: Cleanup" {
        # "#CSM \"Data: Cleanup\"\nCleanup any data and references, here.\n(this is called automatically, by the Macro: Exit)"
        n52 = Unbundle By Name(w183) -> ("Core.Current VI Reference"=w186:refnum<vi>)
        n53 = Close Reference(reference=w186, error in (no error)=w185) -> (error out=w184:errorcluster)
        n54 = call <vilib>:"Add State(s) to Queue__JKI_lib_State_Machine.vi"("State(s) in (\"\")"=w188) -> ("States Out"=w187:string)  [unwired: 14 in]
      }
      frame "---------- UI ----------" {
        # "#CSM \"Category Seperator\"\nDo not put any code in this frame."
        n55 = call <vilib>:"Add State(s) to Queue__JKI_lib_State_Machine.vi"("State(s) in (\"\")"=w193) -> ("States Out"=w192:string)  [unwired: 14 in]
      }
      frame "UI: Initialize" {
        # "#CSM \"UI: Initialize\"\nInitialize the User Interface, here.\n(this is called automatically, by the Macro: Init)"
        n56 = Unbundle By Name(w218) -> ("Sequence Viewer"=w217:refnum<vi>)
        n57 = global read "global-rc-strings.vi" "OI.ErrorDescription(Col4)"() -> (w199:string)
        n58 = global read "global-rc-strings.vi" "OI.TestResult(Col2)"() -> (w197:string)
        n59 = global read "global-rc-strings.vi" "OI.TestStatus(Col3)"() -> (w198:string)
        n60 = global read "global-rc-strings.vi" "OI.StepIndex(Col0)"() -> (w195:string)
        n61 = global read "global-rc-strings.vi" "OI.TestStep(Col1)"() -> (w196:string)
        n62 = Build Array(w195, w196, w197, w198, w199) -> (w194:string[])
        n63 = property class="MCListbox (strict)"(reference=w217, error in=w215, "ItemNames"=string[][] [] ("Item Names"), "Vertical Lines Visible"=TRUE ("Visible Items:Vertical Lines Visible"), "Horizontal Lines Visible"=TRUE ("Visible Items:Horizontal Lines Visible"), "Symbols Vis"=TRUE ("Visible Items:Symbols Visible"), "ColHdrString"=w194, "ActiveCell"=T3 {"Row"=-1, "Column"=-2} ("Active Cell:Active Cell"), "Justify"=enum16{"Left", "Center", "Right"}."Center" ("Active Cell:Cell Justification")) -> (reference out=w207:refnum<vi>, error out=w206:errorcluster)
        n64 = property class="MCListbox (strict)"(reference=w207, error in=w206, "ActiveCell"=T3 {"Row"=-2, "Column"=-2} ("Active Cell:Active Cell"), "CellBG"=u32 16448250) -> (reference out=w205:refnum<vi>, error out=w204:errorcluster)
        n65 = property class="MCListbox (strict)"(reference=w205, error in=w204, "ActiveCell"=T3 {"Row"=-1, "Column"=-2} ("Active Cell:Active Cell"), "CellBG"=u32 15263976) -> (error out=w203:errorcluster)  [unwired: 1 out]
        n66 = call <vilib>:"Add State(s) to Queue__JKI_lib_State_Machine.vi"("State(s) in (\"\")"=w220) -> ("States Out"=w219:string)  [unwired: 14 in]
      }
      frame "UI: Cursor Set" {
        # "Argument"
        # "#CSM \"UI: Cursor Set\"\nSet and Unset Cursor Busy.\n(Usage: \"UI: Cursor Set >> Busy|Idle\")"
        n67 = disable-structure shown="Default" {
          disable-tunnel: w224 -> [w230 w235]
          disable-tunnel: [w229 w235] -> w223
          disable-tunnel: w222 -> [w228 _]
          frame condition #0 (active) {
            n68 = case shown="\"Busy\"" w228 {
              tunnel: w230 -> [w232 w234]
              tunnel: [w231 w233] -> w229
              frame "Idle", Default {
                n69 = call <vilib>:"Unset Busy.vi"("error in (no error)"=w232) -> ("error out"=w231:errorcluster)  [unwired: 10 in]
              }
              frame "Busy" {
                n70 = call <vilib>:"Set Busy.vi"("error in (no error)"=w234) -> ("error out"=w233:errorcluster)  [unwired: 9 in, 1 out]
              }
            }
          }
          frame condition #1 {
          }
        }
        n71 = call <vilib>:"Add State(s) to Queue__JKI_lib_State_Machine.vi"("State(s) in (\"\")"=w227) -> ("States Out"=w226:string)  [unwired: 14 in]
      }
      frame "UI: Front Panel State" {
        # "Argument"
        # "#CSM \"UI: Front Panel State\"\nSet Front Panel Open or Closed\n(Usage: \"UI: Front Panel State >> Open|Close\")"
        n72 = Unbundle By Name(w239) -> ("Core.Current VI Reference"=w238:refnum<vi>)
        n73 = case shown="\"Minimize\", \"Minimized\"" w237 {
          tunnel: w241 -> [w249 w264 w275 w288 w301]
          tunnel: [w251 w265 w277 w290 w303] -> w240
          tunnel: w238 -> [w250 w262 w276 w289 w302]
          frame "Open", "Standard", Default {
            w244 = T1."Standard" ("State")
            n74 = property class="VI"(reference=w250, error in=w249) -> (reference out=w247:refnum<vi>, error out=w248:errorcluster, "FP.State"=w246:T1)
            n75 = Not Equal?(x=w246, y=w244) -> (x != y?=w245:bool)
            n76 = case shown="True" w245 {
              tunnel: [w255 w257] -> w251
              tunnel: w248 -> [w254 w257]
              tunnel: w247 -> [w253 _]
              tunnel: w244 -> [w252 _]
              frame True {
                n77 = invoke class="VI" method="FP.Open"(reference=w253, error in=w254, "Activate"=TRUE, "State"=w252) -> (error out=w255:errorcluster)  [unwired: 1 in, 4 out]
              }
              frame False {
              }
            }
          }
          frame "Close", "Closed" {
            n78 = property class="VI"(reference=w262, error in=w264) -> (reference out=w261:refnum<vi>, error out=w263:errorcluster, "FP.State"=w259:T1)
            n79 = Not Equal?(x=w259, y=T1."Closed" ("Front Panel Window:State")) -> (x != y?=w258:bool)
            n80 = case shown="True" w258 {
              tunnel: [w266 w269] -> w265
              tunnel: w263 -> [w266 w268]
              tunnel: w261 -> [_ w267]
              frame False {
              }
              frame True {
                n81 = invoke class="VI" method="FP.Close"(reference=w267, error in=w268) -> (error out=w269:errorcluster)  [unwired: 1 in, 2 out]
              }
            }
          }
          frame "Hidden", "Hide" {
            w270 = T1."Hidden" ("State")
            n82 = property class="VI"(reference=w276, error in=w275) -> (reference out=w273:refnum<vi>, error out=w274:errorcluster, "FP.State"=w272:T1)
            n83 = Not Equal?(x=w272, y=w270) -> (x != y?=w271:bool)
            n84 = case shown="True" w271 {
              tunnel: [w281 w282] -> w277
              tunnel: w274 -> [w280 w282]
              tunnel: w273 -> [w279 _]
              tunnel: w270 -> [w278 _]
              frame True {
                n85 = invoke class="VI" method="FP.Open"(reference=w279, error in=w280, "State"=w278) -> (error out=w281:errorcluster)  [unwired: 2 in, 4 out]
              }
              frame False {
              }
            }
          }
          frame "Minimize", "Minimized" {
            w283 = T1."Minimized" ("State")
            n86 = property class="VI"(reference=w289, error in=w288) -> (reference out=w286:refnum<vi>, error out=w287:errorcluster, "FP.State"=w285:T1)
            n87 = Not Equal?(x=w285, y=w283) -> (x != y?=w284:bool)
            n88 = case shown="False" w284 {
              tunnel: [w294 w295] -> w290
              tunnel: w287 -> [w293 w295]
              tunnel: w286 -> [w292 _]
              tunnel: w283 -> [w291 _]
              frame True {
                n89 = invoke class="VI" method="FP.Open"(reference=w292, error in=w293, "State"=w291) -> (error out=w294:errorcluster)  [unwired: 2 in, 4 out]
              }
              frame False {
              }
            }
          }
          frame "Maximize", "Maximized" {
            w296 = T1."Maximized" ("State")
            n90 = property class="VI"(reference=w302, error in=w301) -> (reference out=w299:refnum<vi>, error out=w300:errorcluster, "FP.State"=w298:T1)
            n91 = Not Equal?(x=w298, y=w296) -> (x != y?=w297:bool)
            n92 = case shown="True" w297 {
              tunnel: [w307 w308] -> w303
              tunnel: w300 -> [w306 w308]
              tunnel: w299 -> [w305 _]
              tunnel: w296 -> [w304 _]
              frame True {
                n93 = invoke class="VI" method="FP.Open"(reference=w305, error in=w306, "State"=w304) -> (error out=w307:errorcluster)  [unwired: 2 in, 4 out]
              }
              frame False {
              }
            }
          }
        }
        n94 = call <vilib>:"Add State(s) to Queue__JKI_lib_State_Machine.vi"("State(s) in (\"\")"=w243) -> ("States Out"=w242:string)  [unwired: 14 in]
      }
      frame "---------- Macro ----------" {
        # "#CSM \"Category Seperator\"\nDo not put any code in this frame."
        n95 = call <vilib>:"Add State(s) to Queue__JKI_lib_State_Machine.vi"("State(s) in (\"\")"=w313) -> ("States Out"=w312:string)  [unwired: 14 in]
      }
      frame "Macro: Initialize" {
        w315 = "Data: Initialize\nInitialize Core Data\n//Events: Register\nUI: Initialize\n//UI: Front Panel State >> Open"  # Data: Initialize Initialize Core Data //Events: Register UI: Initialize //UI: Front Panel State >> Open
        # "#CSM \"Macro: Initialize\"\nInitialization Macro (This is called once, when the VI starts)"
        n96 = call <vilib>:"Add State(s) to Queue__JKI_lib_State_Machine.vi"("State(s) in Front (\"\")"=w315, "State(s) in (\"\")"=w319) -> ("States Out"=w318:string)  [unwired: 13 in]
      }
      frame "Macro: Exit" {
        # "#CSM \"Macro: Exit\"\nExit Macro (This is called once, when the VI exits)"
        n97 = Unbundle By Name(w328) -> ("Core.Close Panel on Exit?"=w327:bool)
        n98 = Select(t="UI: Front Panel State >> Close", s=w327, f="") -> (s? t:f=w324:string)
        n99 = call <vilib>:"Add State(s) to Queue__JKI_lib_State_Machine.vi"("State(s) in Front (\"\")"="//Exit Sub-Modules ", "State(s) in (\"\")"=w324, "State(s) at Back (\"\")"="Data: Cleanup\n//Events: Unregister\nExit") -> ("States Out"=w322:string)  [unwired: 12 in]
        n100 = call <vilib>:"Add State(s) to Queue__JKI_lib_State_Machine.vi"("State(s) in Front (\"\")"=w322, "State(s) in (\"\")"=w331) -> ("States Out"=w330:string)  [unwired: 13 in]
      }
      frame "---------- API ----------" {
        # "#CSM \"Category Seperator\"\nDo not put any code in this frame."
      }
      frame "TS: Load Sequence" {
        # "#CSM API Example\nCopy/Rename this case for your own API"
        n101 = Unbundle By Name(w348) -> ("Sequence Viewer"=w347:refnum<vi>, "Core.Current VI Reference"=w339:refnum<vi>)
        n102 = call "Argument to Large String.vi"("Arguments"=w344) -> ("error out"=w336:errorcluster, "String"=w346:string)  [unwired: 9 in]
        n103 = call <userlib>:"Defer Panel Updates_csm.vi"("Error In"=w336, "Defer Updates?"=TRUE, "VI Reference (Caller)"=w339) -> ("Error Out"=w342:errorcluster, "VI Reference (Caller) 2"=w340:refnum<vi>)  [unwired: 7 in]
        n104 = call "Sequence-Load.vi"("error in (no error)"=w342, "Sequence String"=w346, "MCListbox Refnum"=w347) -> ("error out"=w345:errorcluster)  [unwired: 7 in, 1 out]
        n105 = call <userlib>:"Defer Panel Updates_csm.vi"("Error In"=w345, "Defer Updates?"=FALSE, "VI Reference (Caller)"=w340) -> ("Error Out"=w341:errorcluster)  [unwired: 7 in, 1 out]
        n106 = call <vilib>:"Add State(s) to Queue__JKI_lib_State_Machine.vi"("State(s) in (\"\")"=w350) -> ("States Out"=w349:string)  [unwired: 14 in]
      }
      frame "TS: Link to Engine" {
        w353 = "//Connect UI With Engine\nSequenceLoaded Event@<1> >>TS: Load Sequence -><register> \nSequenceUnloaded Event@<1> >> TS: Load Sequence -><register> \nTestStarted Event@<1> >>TS: Test Started Handler -><register> \nStepComplete Event@<1> >>TS: Step Complete Handler -><register> \nTestComplete Event@<1> >>TS: Test Complete Handler -><register> \nTestTerminated Event@<1> >>TS: Test Complete Handler -><register>\nStepStart Event@<1> >>TS: Step Start Handler -><register> "  # //Connect UI With Engine SequenceLoaded Event@<1> >>TS: Load Sequence -><register>  SequenceUnloaded Event@<1> >> TS: Load Sequence -><register>  TestStarted Event@<1> >>TS: Test Started Handler -><register>  StepComplete Event@<1> >>TS: Step Complete Handler -><register>  TestComplete Event@<1> >>TS: Test Complete Handler -><register>  TestTerminated Event@<1> >>TS: Test Complete Handler -><register> StepStart Event@<1> >>TS: Step Start Handler -><register>
        n107 = call-poly <userlib>:"Build Message with Arguments++.vi"("States With Replace Token"=w353, "<1>"=w351) -> ("States"=w352:string)  [unwired: 13 in]
        n108 = call <vilib>:"Add State(s) to Queue__JKI_lib_State_Machine.vi"("State(s) in Front (\"\")"=w352, "State(s) in (\"\")"=w354) -> ("States Out"=w355:string)  [unwired: 13 in]
      }
      frame "TS: Test Started Handler" {
        # "#CSM API Example\nCopy/Rename this case for your own API"
        n109 = Unbundle By Name(w359) -> ("Sequence Viewer"=w358:refnum<vi>, "Core.Current VI Reference"=w366:refnum<vi>)
        n110 = call <userlib>:"Defer Panel Updates_csm.vi"("Error In"=w360, "Defer Updates?"=TRUE, "VI Reference (Caller)"=w366) -> ("Error Out"=w363:errorcluster, "VI Reference (Caller) 2"=w367:refnum<vi>)  [unwired: 7 in]
        n111 = call "Sequence-Started.vi"("error in (no error)"=w363, "MCListbox Refnum"=w358) -> ("error out"=w362:errorcluster)  [unwired: 8 in, 1 out]
        n112 = call <userlib>:"Defer Panel Updates_csm.vi"("Error In"=w362, "Defer Updates?"=FALSE, "VI Reference (Caller)"=w367) -> ("Error Out"=w361:errorcluster)  [unwired: 7 in, 1 out]
        n113 = call <vilib>:"Add State(s) to Queue__JKI_lib_State_Machine.vi"("State(s) in (\"\")"=w370) -> ("States Out"=w369:string)  [unwired: 14 in]
      }
      frame "TS: Step Start Handler" {
        # "#CSM API Example\nCopy/Rename this case for your own API"
        n114 = Unbundle By Name(w374) -> ("Sequence Viewer"=w373:refnum<vi>, "Core.Current VI Reference"=w378:refnum<vi>)
        n115 = call <userlib>:"Defer Panel Updates_csm.vi"("Defer Updates?"=TRUE, "VI Reference (Caller)"=w378) -> ("Error Out"=w372:errorcluster, "VI Reference (Caller) 2"=w379:refnum<vi>)  [unwired: 8 in]
        n116 = call "Convert API String Arguments to Data.vim"("Reference Type"=T4 {"index"=0, "Response"="", "error"={"status"=FALSE, "code"=0, "source"=""}} ("StepComplete Event Data"), "error in (no error)"=w372, "API String"=w382) -> ("error out"=w383:errorcluster, "Data"=w381:T4)  [unwired: 5 in]
        n117 = call "Sequence-StepStart.vi"("MCListbox Refnum"=w373, "Step Feedback"=w381, "error in (no error)"=w383) -> ("error out"=w371:errorcluster)  [unwired: 11 in, 1 out]
        n118 = call <userlib>:"Defer Panel Updates_csm.vi"("Error In"=w371, "Defer Updates?"=FALSE, "VI Reference (Caller)"=w379) -> ("Error Out"=w375:errorcluster)  [unwired: 7 in, 1 out]
      }
      frame "TS: Step Complete Handler" {
        # "#CSM API Example\nCopy/Rename this case for your own API"
        n119 = Unbundle By Name(w386) -> ("Core.Current VI Reference"=w392:refnum<vi>)
        n120 = Unbundle By Name(w386) -> ("Sequence Viewer"=w400:refnum<vi>, "ResponseMaxLen"=w394:i32)
        n121 = call <userlib>:"Defer Panel Updates_csm.vi"("Defer Updates?"=TRUE, "VI Reference (Caller)"=w392) -> ("Error Out"=w389:errorcluster, "VI Reference (Caller) 2"=w393:refnum<vi>)  [unwired: 8 in]
        n122 = call "Convert API String Arguments to Data.vim"("Reference Type"=T4 {"index"=0, "Response"="", "error"={"status"=FALSE, "code"=0, "source"=""}} ("StepComplete Event Data"), "error in (no error)"=w389, "API String"=w397) -> ("error out"=w398:errorcluster, "Data"=w396:T4)  [unwired: 5 in]
        n123 = call "Sequence-StepComplete.vi"("MCListbox Refnum"=w400, "Step Feedback"=w396, "error in (no error)"=w398, "length (rest)"=w394) -> ("error out"=w388:errorcluster)  [unwired: 10 in, 1 out]
        n124 = call <userlib>:"Defer Panel Updates_csm.vi"("Error In"=w388, "Defer Updates?"=FALSE, "VI Reference (Caller)"=w393) -> ("Error Out"=w387:errorcluster)  [unwired: 7 in, 1 out]
      }
      frame "TS: Test Complete Handler" {
        # "#CSM API Example\nCopy/Rename this case for your own API"
      }
      frame "---------- Internal ----------" {
        # "#CSM \"Category Seperator\"\nDo not put any code in this frame."
        n125 = call <vilib>:"Add State(s) to Queue__JKI_lib_State_Machine.vi"("State(s) in (\"\")"=w410) -> ("States Out"=w409:string)  [unwired: 14 in]
      }
      frame "Internal: action1" {
        # "#CSM \"Internal State\"\nThis category is used for holding internal states"
        n126 = call <vilib>:"Add State(s) to Queue__JKI_lib_State_Machine.vi"("State(s) in (\"\")"=w415) -> ("States Out"=w414:string)  [unwired: 14 in]
      }
      frame "Internal: action2" {
        # "#CSM \"Internal State\"\nThis category is used for holding internal states"
        n127 = call <vilib>:"Add State(s) to Queue__JKI_lib_State_Machine.vi"("State(s) in (\"\")"=w420) -> ("States Out"=w419:string)  [unwired: 14 in]
      }
    }
  }
